vi "PID Derivative Action (DBL Array).vi"(4 "dt (min)":dbl format="%.3f", 5 "initialize (F)":bool, 6 "Kd":dbl[](array[numeric]) format="%.2f", 7 "process variable":dbl[](array[numeric]) format="%.2f") -> (3 "derivative action":dbl[](array[numeric]) format="%.2f")   [LabVIEW 2020, in "NI_PID_pid.lvlib"]
uses:
  <vilib>/addons/control/pid/NI_PID_pid.lvlib
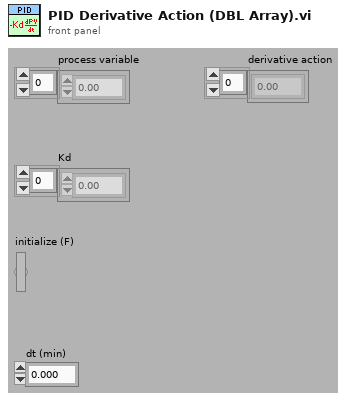
[diagram p1: front panel]
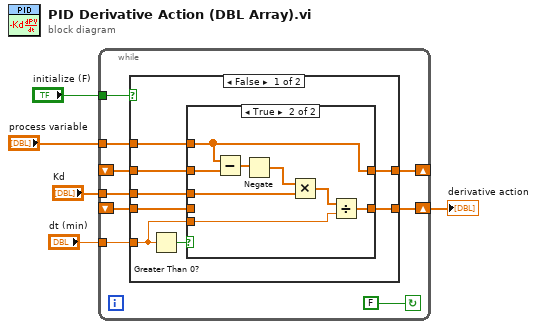
[diagram p0: block diagram]
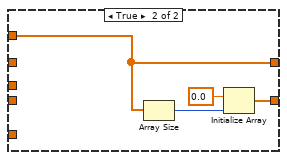
[diagram p3: hidden frame]
diagram:
  n1 = while {
    tunnel: "Kd" -> [w8]
    shift-left: _ -> [w9]
    shift-right: [w7] -> w1
    tunnel: "process variable" -> [w12]
    shift-left: _ -> [w11]
    shift-right: [w10] -> _
    tunnel: "dt (min)" -> [w13]
    tunnel: "initialize (F)" -> [w14]
    stop <- FALSE continue-if-true
    n2 = case shown="False" w14 {
      tunnel: w11 -> [w22 _]
      tunnel: w8 -> [w19 _]
      tunnel: w12 -> [w21 w36]
      tunnel: [w18 w36] -> w10
      tunnel: [w20 w34] -> w7
      tunnel: w9 -> [w16 _]
      tunnel: w13 -> [w15 _]
      frame False {
        n3 = Greater Than 0?(x=w15) -> (x > 0?=w17:bool)
        n4 = case shown="True" w17 {
          tunnel: w22 -> [w24 w30]
          tunnel: w15 -> [_ w29]
          tunnel: w21 -> [_ w25]
          tunnel: [w23 w28] -> w20
          tunnel: w19 -> [_ w26]
          tunnel: [w24 w25] -> w18
          tunnel: w16 -> [w23 _]
          frame False {
            # "dt = 0 min"
          }
          frame True {
            n5 = Subtract(x=w25, y=w30) -> (x-y=w32:dbl[])
            n6 = Negate(x=w32) -> (-x=w27:dbl[])
            n7 = Multiply(x=w27, y=w26) -> (x*y=w31:dbl[])
            n8 = Divide(x=w31, y=w29) -> (x/y=w28:dbl[])
          }
        }
      }
      frame True {
        n9 = Array Size(array=w36) -> (size(s)=w35:i32)
        n10 = Initialize Array(0.0 ("Element Data"), w35) -> (w34:dbl[])
      }
    }
  }
  "derivative action" <- w1
